vi "AlazarEngine.vi"(0 "Device ID":T4={"System ID"=1, "Board ID"=1}, 1 "Capture Clock":T3={"Sample Rate"=30, "Decimation"=0, "Source"=1, "Edge"=0} {"Edge" items=["Rising", "Falling"]; "Source" items=["Internal"=1, "Fast External"=2, "Medium External"=3, "Slow External"=4, "External AC"=5, "External DC"=6, "External 10MHz"=7]}, 2 "Ch Input Control":T5={"Channel"=1, "Coupling"=2, "Range"=10, "Impedance"=2} {"Channel" items=["A"=1, "B"=2, "C"=4, "D"=8]; "Coupling" items=["AC"=1, "DC"=2]; "Range" items=["20 mV"=1, "40 mV"=2, "50 mV"=3, "80 mV"=4, "100 mV"=5, "200 mV"=6, "400 mV"=7, "500 mV"=8, "800 mV"=9, "1 V"=10, "1.25 V"=33, "2 V"=11, "4 V"=12, "5 V"=13, "8 V"=14, "10 V"=15, "20 V"=16]; "Impedance" items=["1 MOhm"=1, "50 Ohm"=2, ""=0]}, 3 "Acq Settings":T1={"Record Length"=1536, "Offset"=0, "Records Per Buffer"=1000, "Records Count (Records/Acq)"=2147483647, "Window Type"=1, "Footer"=0, "Samples per record"=2048, "Output Format"=257} {"Output Format" items=["Float Log"=11, "Float Amp"=10, "U16_LOG"=1, "U16_AMP2"=257, "Real"=3, "Imag"=4]; "Footer" items=["FOOTER_NONE", "FOOTER_NPT"]; "Window Type" items=["DSP_WINDOW_NONE", "DSP_WINDOW_HANNING", "DSP_WINDOW_HAMMING", "DSP_WINDOW_BLACKMAN", "DSP_WINDOW_BLACKMAN_HARRIS", "DSP_WINDOW_BARTLETT"]}, 4 "Trigger Settings":T8={"General Trigger Settings"={"Trigger Operation"=0, "Coupling ID"=2, "Range ID"=0, "Delay"=0, "Timeout Ticks"=0, "Mode"=0, "Parameter"=0}, "Trigger Engine 1"={"Trigger Engine"=0, "Source"=0, "Slope"=1, "Level"=0}, "Trigger Engine 2"={"Trigger Engine"=0, "Source"=0, "Slope"=1, "Level"=0}} {"General Trigger Settings"."Trigger Operation" items=["J", "K", "J OR K", "J AND K", "J XOR K", "J AND NOT K", "NOT J AND K"]; "General Trigger Settings"."Coupling ID" items=["AC"=1, "DC"=2]; "General Trigger Settings"."Range ID" items=["5 V", "1 V", "TTL"]; "Trigger Engine 1"."Trigger Engine" items=["J", "K"]; "Trigger Engine 1"."Source" items=["A", "B", "External", "Disable", "C", "D"]; "Trigger Engine 1"."Slope" items=["Positive"=1, "Negative"=2]; "Trigger Engine 2"."Trigger Engine" items=["J", "K"]; "Trigger Engine 2"."Source" items=["A", "B", "External", "Disable", "C", "D"]; "Trigger Engine 2"."Slope" items=["Positive"=1, "Negative"=2]}, 5 "error in (no error)":errorcluster, 6 "Action":T2=enum."Config Trig", 9 "Imag window array":sgl[](array[numeric]), 10 "FFT Channel":u32(ring)=1 items=["A"=1, "B"=2, "A + B"=3, "C"=4, "A + C"=5, "A + B"=6, "D"=8, "A + D"=9, "B + D"=10, "C + D"=12, "A + B + C + D"=15]) -> (14 "FFT Buffer":sgl[](array[numeric]), 15 "Buffer":u16[](array[numeric]), 19 "error out":errorcluster)   [LabVIEW 2018]
uses:
  Controls/General Trigger Settings.ctl
  Controls/Trigger Engine Controls.ctl
  Controls/Channel Input Controls.ctl
  Controls/Alazar Device ID.ctl
  Controls/Clock Controls.ctl
  Controls/Alazar Engine Actions.ctl
  Controls/Alazar Acquisition Settings.ctl
  Controls/Async Read Parameters.ctl
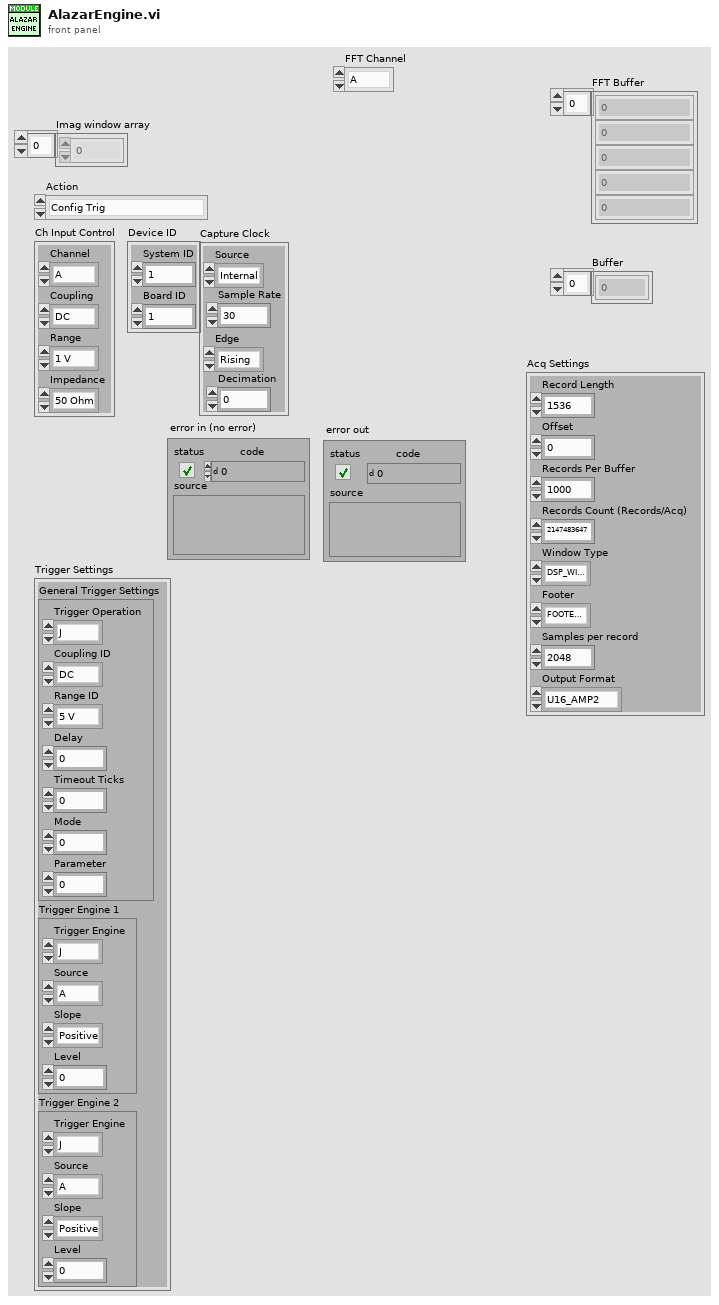
[diagram p1: front panel]
types:
  T1 = typedef "Alazar Acquisition Settings.ctl" = cluster{"Record Length":u32, "Offset":u32, "Records Per Buffer":u32, "Records Count (Records/Acq)":u32, "Window Type":u32, "Footer":u32, "Samples per record":u32, "Output Format":u32}
  T2 = typedef "Alazar Engine Actions.ctl" = enum16{"Init", "Config Clock", "Config Ch", "Config Trig", "Config Non-FFT Acq.", "Non-FFT Acquire", "start acquire", "Config Acq.", "Acquire", "UnInit"}
  T3 = typedef "Clock Controls.ctl" = cluster{"Sample Rate":u32, "Decimation":u32, "Source":u32, "Edge":u32}
  T4 = typedef "Alazar Device ID.ctl" = cluster{"System ID":u32, "Board ID":u32}
  T5 = typedef "Channel Input Controls.ctl" = cluster{"Channel":u8, "Coupling":u32, "Range":u32, "Impedance":u32}
  T6 = typedef "General Trigger Settings.ctl" = cluster{"Trigger Operation":u32, "Coupling ID":u32, "Range ID":u32, "Delay":u32, "Timeout Ticks":u32, "Mode":u32, "Parameter":u32}
  T7 = typedef "Trigger Engine Controls.ctl" = cluster{"Trigger Engine":u32, "Source":u32, "Slope":u32, "Level":u32}
  T8 = cluster{"General Trigger Settings":T6, "Trigger Engine 1":T7, "Trigger Engine 2":T7}
  T9 = typedef "Async Read Parameters.ctl" = cluster{"Transfer Offset":u32, "Transfer Length":u32, "Records Per Buffer":u32, "Records Per Acquisition":u32}
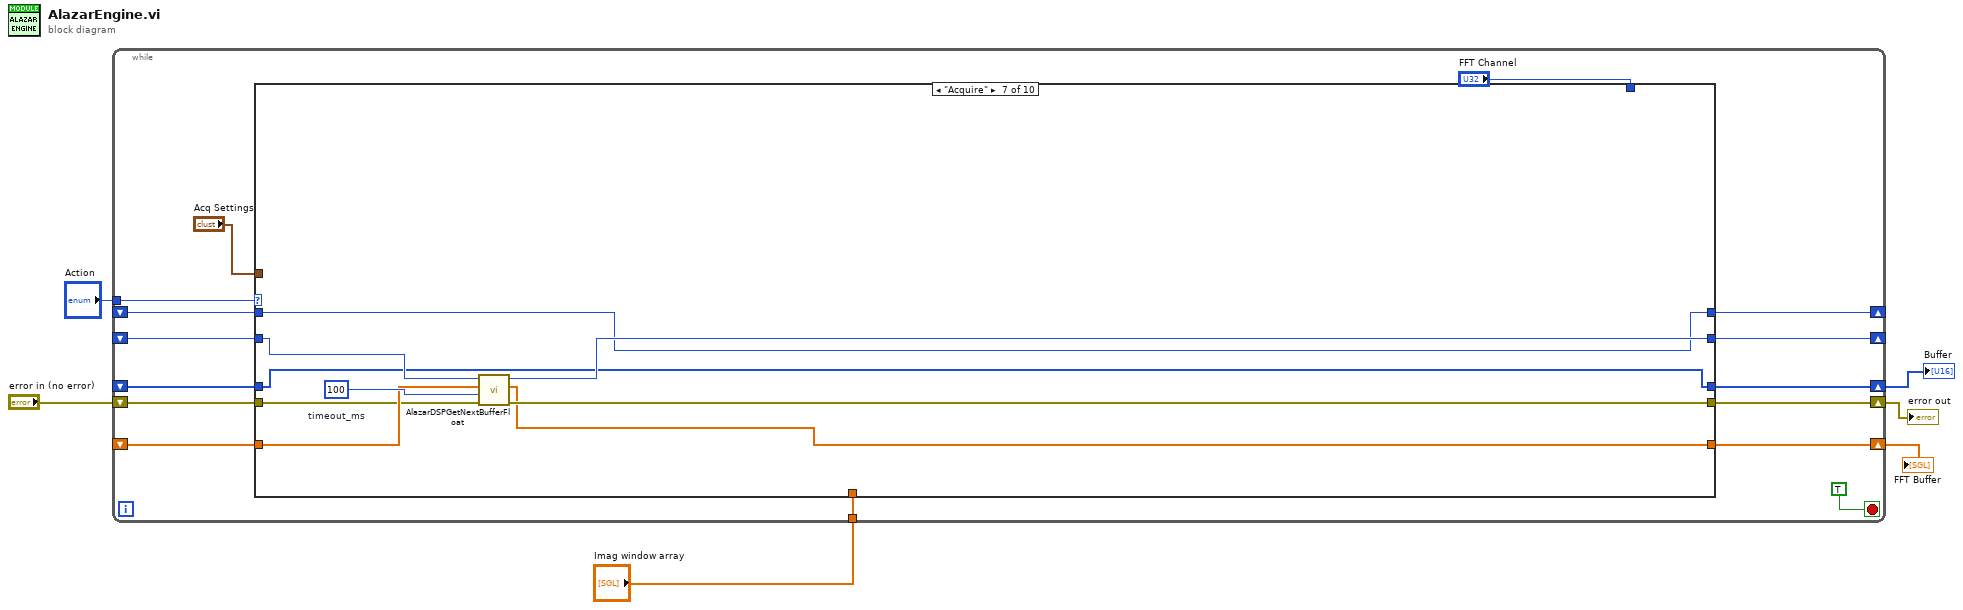
[diagram p0: block diagram]
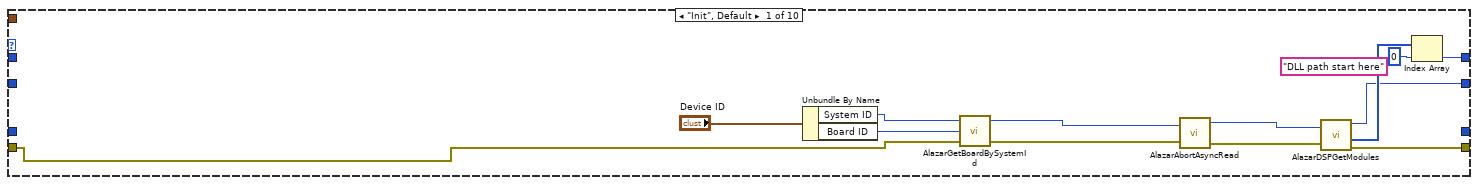
[diagram p2: hidden frame]
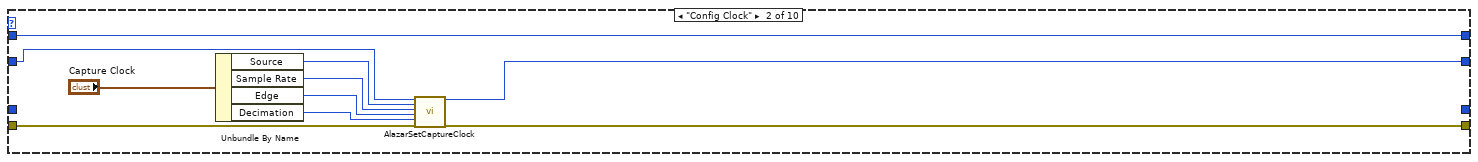
[diagram p3: hidden frame]
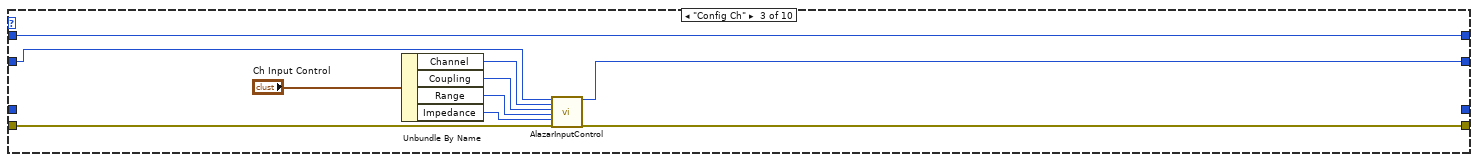
[diagram p4: hidden frame]
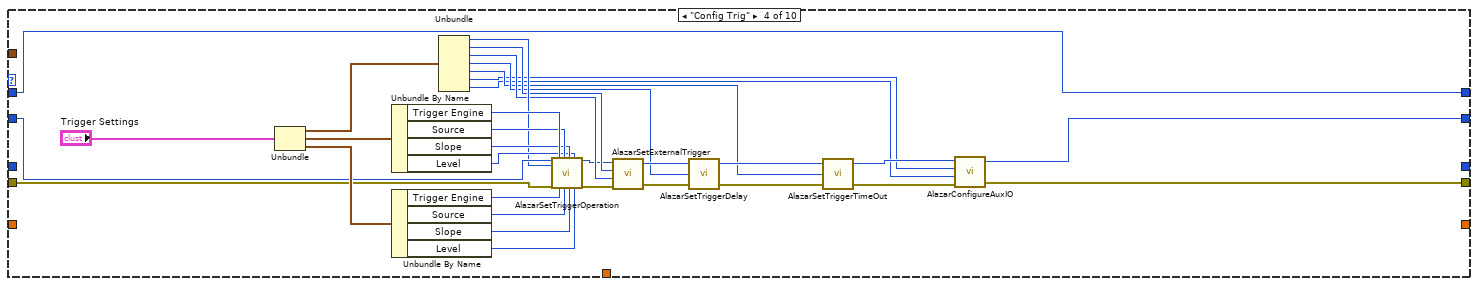
[diagram p5: hidden frame]
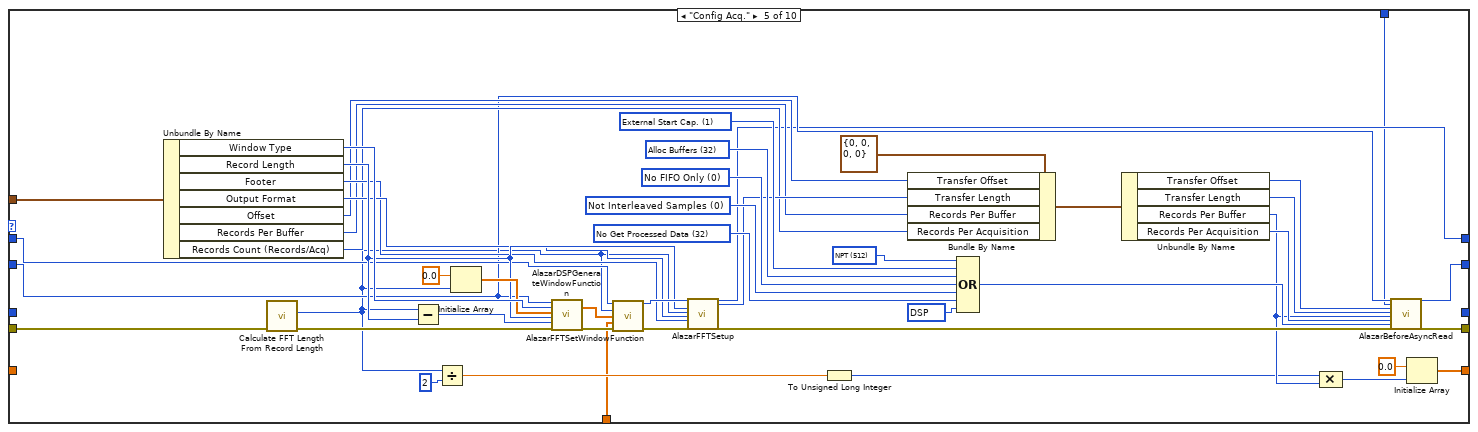
[diagram p6: hidden frame]
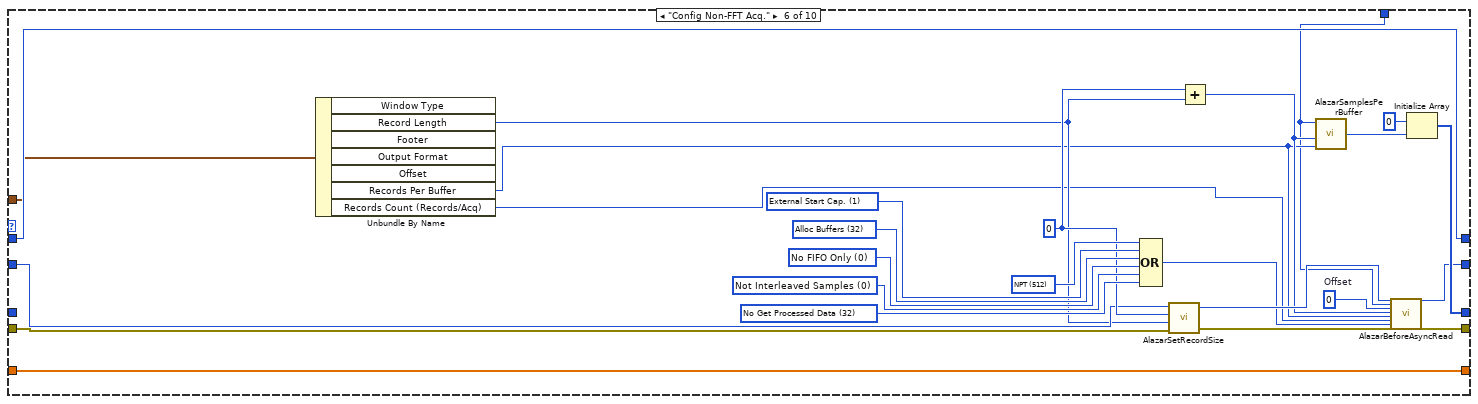
[diagram p7: hidden frame]
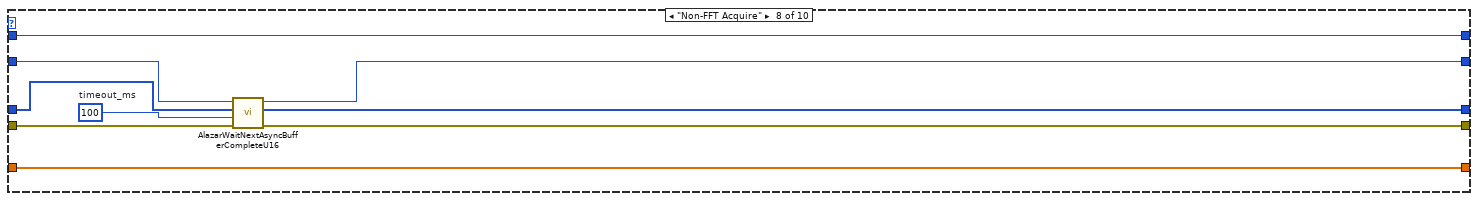
[diagram p8: hidden frame]
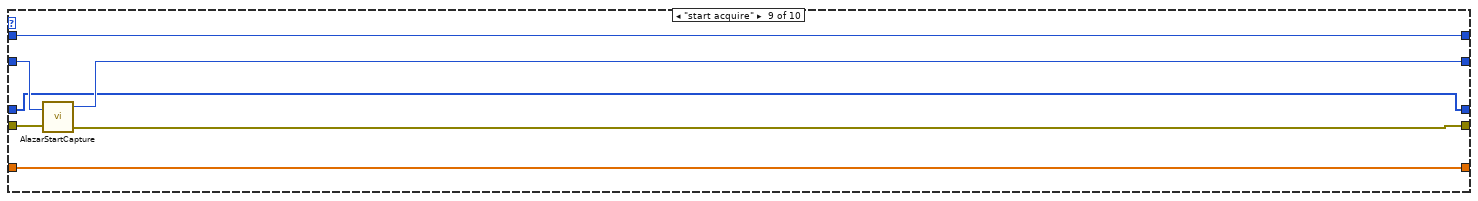
[diagram p9: hidden frame]
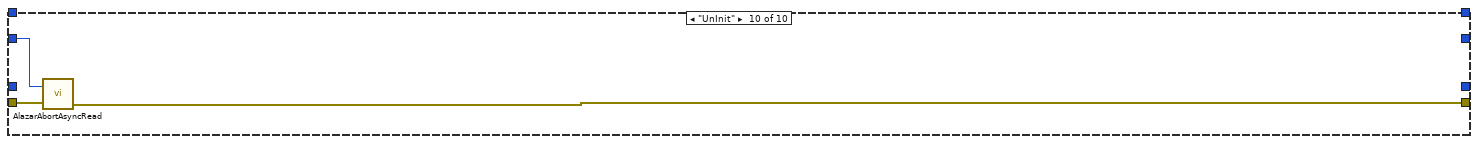
[diagram p10: hidden frame]
diagram:
  n1 = while {
    tunnel: "Action" -> [w19]
    shift-right: [w18] -> _
    shift-left: _ -> [w17]
    shift-right: [w16] -> _
    shift-left: _ -> [w15]
    shift-right: [w14] -> w4
    shift-left: "error in (no error)" -> [w20]
    shift-right: [w13] -> w3
    shift-left: _ -> [w12]
    shift-right: [w11] -> w1
    shift-left: _ -> [w10]
    tunnel: "Imag window array" -> [w9]
    stop <- TRUE stop-if-true
    n2 = case shown="\"Acquire\"" w19 {
      tunnel: w20 -> [w22 w42 w48 w68 w125 w145 w163 w174 w184 w187]
      tunnel: [w25 w35 w47 w56 w90 w144 w162 w170 w183 w185] -> w14
      tunnel: [w23 w36 w46 w55 w101 w139 w167 w172 w181 _] -> w18
      tunnel: w17 -> [_ w37 w45 w73 w106 w141 w168 w175 w182 w186]
      tunnel: [w33 w44 w54 w84 w99 w140 w166 w173 w180 _] -> w16
      tunnel: w15 -> [_ w44 w54 w84 w113 w140 w166 w173 w180 _]
      tunnel: [_ _ _ _ w92 w142 w161 w171 w179 _] -> w13
      tunnel: w12 -> [_ _ _ _ _ w142 w164 w171 w179 _]
      tunnel: [_ _ _ _ _ w143 w160 w169 w178 _] -> w11
      tunnel: w10 -> [_ _ _ _ _ _ w160 w176 w178 _]
      tunnel: w9 -> [_ _ _ _ w89 _ _ _ _ _]
      tunnel: "Acq Settings" -> [_ _ _ _ w88 w138 _ _ _ _]
      tunnel: "FFT Channel" -> [_ _ _ _ w87 w134 _ _ _ _]
      frame "Init", Default {
        (unwired) "DLL path start here"
        n3 = Unbundle By Name("Device ID") -> ("System ID"=w31:u32, "Board ID"=w30:u32)
        n4 = call "AlazarGetBoardBySystemId.vi"("error in (no error)"=w22, "Board ID"=w30, "System ID"=w31) -> ("error out"=w29:errorcluster, "Handle"=w28:u64)  [unwired: 1 out]
        n5 = call "AlazarAbortAsyncRead.vi"("Handle"=w28, "error in (no error)"=w29) -> ("Handle"=w27:u64, "error out"=w26:errorcluster)  [unwired: 1 out]
        n6 = call "AlazarDSPGetModules.vi"("Handle"=w27, "error in (no error)"=w26) -> ("Handle"=w23:u64, "DSP Modules"=w24:u64[], "error out"=w25:errorcluster)  [unwired: 1 out]
        n7 = Index Array(array=w24, index=u32 0) -> (element=w33:u64)
      }
      frame "Config Clock" {
        n8 = Unbundle By Name("Capture Clock") -> ("Source"=w38:u32, "Sample Rate"=w39:u32, "Edge"=w40:u32, "Decimation"=w41:u32)
        n9 = call "AlazarSetCaptureClock.vi"("Handle"=w37, "Source"=w38, "Sample Rate"=w39, "Edge"=w40, "Decimation"=w41, "error in (no error)"=w42) -> ("Handle"=w36:u64, "error out"=w35:errorcluster)  [unwired: 11 in, 1 out]
      }
      frame "Config Ch" {
        n10 = Unbundle By Name("Ch Input Control") -> ("Channel"=w52:u8, "Coupling"=w51:u32, "Range"=w50:u32, "Impedance"=w49:u32)
        n11 = call "AlazarInputControl.vi"("Handle"=w45, "Channel"=w52, "Coupling"=w51, "Range"=w50, "Impedance"=w49, "error in (no error)"=w48) -> ("Handle"=w46:u64, "error out"=w47:errorcluster)  [unwired: 11 in, 1 out]
      }
      frame "Config Trig" {
        n12 = Unbundle("Trigger Settings") -> ("General Trigger Settings"=w85:T6, "Trigger Engine 1"=w83:T7, "Trigger Engine 2"=w82:T7)
        n13 = Unbundle By Name(w83) -> ("Trigger Engine"=w81:u32, "Source"=w80:u32, "Slope"=w79:u32, "Level"=w78:u32)
        n14 = Unbundle By Name(w82) -> ("Trigger Engine"=w77:u32, "Source"=w76:u32, "Slope"=w75:u32, "Level"=w74:u32)
        n15 = Unbundle(w85) -> ("Trigger Operation"=w72:u32, "Coupling ID"=w71:u32, "Range ID"=w70:u32, "Delay"=w64:u32, "Timeout Ticks"=w61:u32, "Mode"=w58:u32, "Parameter"=w57:u32)
        n16 = call "AlazarSetTriggerOperation.vi"("Handle"=w73, "Trigger Operation"=w72, "error in (no error)"=w68, "Trigger Engine 1"=w81, "Trigger Engine 2"=w77, "Source 1"=w80, "Source 2"=w76, "Slope 1"=w79, "Slope 2"=w75, "Level 1"=w78, "Level 2"=w74) -> ("Handle"=w66:u64, "error out"=w69:errorcluster)  [unwired: 6 in, 1 out]
        n17 = call "AlazarSetExternalTrigger.vi"("error in (no error)"=w69, "Range ID"=w70, "Coupling ID"=w71, "Handle"=w66) -> ("error out"=w67:errorcluster, "Handle"=w65:u64)  [unwired: 1 out]
        n18 = call "AlazarSetTriggerDelay.vi"("error in (no error)"=w67, "Delay"=w64, "Handle"=w65) -> ("error out"=w63:errorcluster, "Handle"=w62:u64)  [unwired: 1 out]
        n19 = call "AlazarSetTriggerTimeOut.vi"("error in (no error)"=w63, "Timeout Ticks"=w61, "Handle"=w62) -> ("error out"=w60:errorcluster, "Handle"=w59:u64)  [unwired: 1 out]
        n20 = call "AlazarConfigureAuxIO.vi"("error in (no error)"=w60, "Parameter"=w57, "Mode"=w58, "Handle"=w59) -> ("error out"=w56:errorcluster, "Handle"=w55:u64)  [unwired: 1 out]
      }
      frame "Config Acq." {
        w126 = u32 16384 items=["DSP"=16384]
        w132 = u32 32 items=["No Get Processed Data"=32, "Get Processed Data"=8192]
        w131 = u32 0 items=["Not Interleaved Samples"=0, "Interleave Samples"=4096]
        w127 = u32 0 items=["No FIFO Only"=0, "FIFO Only"=2048]
        w130 = u32 32 items=["Alloc Buffers"=32]
        w129 = u32 1 items=["Internal Start Cap.", "External Start Cap."]
        w128 = u32 512 items=["Traditional"=0, "NPT"=512, "Continuous"=256, "Triggered Streaming"=1024]
        n21 = Unbundle By Name(w88) -> ("Window Type"=w123:u32, "Record Length"=w117:u32, "Footer"=w115:u32, "Output Format"=w116:u32, "Offset"=w111:u32, "Records Per Buffer"=w109:u32, "Records Count (Records/Acq)"=w108:u32)
        n22 = call "Calculate FFT Length From Record Length.vi"("error in (no error)"=w125) -> ("error out"=w124:errorcluster, "FFT Length"=w97:u32)  [unwired: 8 in, 1 out]
        n23 = Subtract(x=w97, y=w117) -> (x-y=w122:u32)
        n24 = Divide(x=w97, y=u32 2) -> (x/y=w93:dbl)
        n25 = Initialize Array(sgl 0.0, w97) -> (w120:sgl[])
        n26 = call "AlazarDSPGenerateWindowFunction.vi"("Handle"=w106, "Window Type"=w123, "window"=w120, "WindowLength_samples"=w117, "PaddingLength_samples"=w122, "error in (no error)"=w124) -> ("window"=w121:sgl[], "error out"=w119:errorcluster)  [unwired: 10 in, 2 out]
        n27 = call "AlazarFFTSetWindowFunction.vi"("DSP Handle"=w113, "Samples per record"=w97, "Real window array"=w121, "Imag window array"=w89, "error in (no error)"=w119) -> ("DSP Handle"=w118:u64, "error out"=w114:errorcluster)  [unwired: 9 in]
        n28 = call "AlazarFFTSetup.vi"("DSP Handle"=w118, "Record Length (samples)"=w117, "FFT Length (samples)"=w97, "Output Format"=w116, "Footer"=w115, "error in (no error)"=w114) -> ("DSP Handle"=w99:u64, "Bytes Per Output Record"=w110:u32, "error out"=w100:errorcluster)  [unwired: 18 in, 1 out]
        n29 = To Unsigned Long Integer(number=w93) -> (unsigned 32bit integer=w91:u32)
        n30 = Bundle By Name(cluster=T9 {"Transfer Offset"=0, "Transfer Length"=0, "Records Per Buffer"=0, "Records Per Acquisition"=0} ("ASync Read Parameters"), "Transfer Offset"=w111, "Transfer Length"=w110, "Records Per Buffer"=w109, "Records Per Acquisition"=w108) -> (w107:T9)
        n31 = Compound Arithmetic op=OR(w128, w129, w130, w127, w131, w132, w126) -> (w102:u32)
        n32 = Unbundle By Name(w107) -> ("Transfer Offset"=w105:u32, "Transfer Length"=w104:u32, "Records Per Buffer"=w98:u32, "Records Per Acquisition"=w103:u32)
        n33 = Compound Arithmetic op=MULTIPLY(w91, w98) -> (w96:u32)
        n34 = call "AlazarBeforeAsyncRead.vi"("Handle"=w106, "Channel Select"=w87, "Transfer Offset"=w105, "Transfer Length"=w104, "Records Per Buffer"=w98, "Records Per Acquisition"=w103, "Flags"=w102, "error in (no error)"=w100) -> ("Handle"=w101:u64, "error out"=w90:errorcluster)  [unwired: 17 in, 1 out]
        n35 = Initialize Array(sgl 0.0 ("element"), w96) -> (w92:sgl[])
      }
      frame "Config Non-FFT Acq." {
        w149 = u32 0  # Offset
        w153 = u32 0 ("Pre-trigger Samples")
        w159 = u32 32 items=["No Get Processed Data"=32, "Get Processed Data"=8192]
        w158 = u32 0 items=["Not Interleaved Samples"=0, "Interleave Samples"=4096]
        w154 = u32 0 items=["No FIFO Only"=0, "FIFO Only"=2048]
        w157 = u32 32 items=["Alloc Buffers"=32]
        w156 = u32 1 items=["Internal Start Cap.", "External Start Cap."]
        w155 = u32 512 items=["Traditional"=0, "NPT"=512, "Continuous"=256, "Triggered Streaming"=1024]
        n36 = Unbundle By Name(w138) -> ("Record Length"=w137:u32, "Records Per Buffer"=w136:u32, "Records Count (Records/Acq)"=w135:u32)  [unwired: 4 out]
        n37 = Compound Arithmetic op=OR(w155, w156, w157, w154, w158, w159) -> (w150:u32)
        n38 = call "AlazarSetRecordSize.vi"("error in (no error)"=w145, "Post-trigger Samples"=w137, "Pre-trigger Samples"=w153, "Handle"=w141) -> ("error out"=w151:errorcluster, "Handle"=w152:u64)  [unwired: 1 out]
        n39 = Add(x=w153, y=w137) -> (x+y=w146:u32)
        n40 = call "AlazarSamplesPerBuffer.vi"("Records Per Buffer"=w136, "Samples Per Record"=w146, "Channel Mask"=w134) -> ("Samples Per Buffer"=w147:u32)  [unwired: 1 in]
        n41 = call "AlazarBeforeAsyncRead.vi"("Handle"=w152, "Channel Select"=w134, "Transfer Offset"=w149, "Transfer Length"=w146, "Records Per Buffer"=w136, "Records Per Acquisition"=w135, "Flags"=w150, "error in (no error)"=w151) -> ("Handle"=w139:u64, "error out"=w144:errorcluster)  [unwired: 17 in, 1 out]
        n42 = Initialize Array(u16 0, w147) -> (w143:u16[])
      }
      frame "Acquire" {
        w165 = u32 100  # timeout_ms
        n43 = call "AlazarDSPGetNextBufferFloat.vi"("error in (no error)"=w163, "timeout_ms"=w165, "Buffer"=w164, "Handle"=w168) -> ("error out"=w162:errorcluster, "Buffer"=w161:sgl[], "Handle"=w167:u64)  [unwired: 1 out]
      }
      frame "Non-FFT Acquire" {
        w177 = u32 100  # timeout_ms
        n44 = call "AlazarWaitNextAsyncBufferCompleteU16.vi"("error in (no error)"=w174, "Timeout (ms)"=w177, "Buffer"=w176, "Handle"=w175) -> ("error out"=w170:errorcluster, "Buffer"=w169:u16[], "Handle"=w172:u64)  [unwired: 1 out]
      }
      frame "start acquire" {
        n45 = call "AlazarStartCapture.vi"("Handle"=w182, "error in (no error)"=w184) -> ("Handle"=w181:u64, "error out"=w183:errorcluster)  [unwired: 1 out]
      }
      frame "UnInit" {
        n46 = call "AlazarAbortAsyncRead.vi"("Handle"=w186, "error in (no error)"=w187) -> ("error out"=w185:errorcluster)  [unwired: 2 out]
      }
    }
  }
  "error out" <- w4
  "FFT Buffer" <- w3
  "Buffer" <- w1
